vi "Configure Subnet Mask.vi"(0 "VISA resource name":refnum<visa-resource-name>, 5 "Subnet Mask (255.255.255.0)":string="255.255.255.0", 11 "error in (no error)":errorcluster) -> (4 "VISA resource name out":refnum<visa-resource-name>, 15 "error out":errorcluster)   [LabVIEW 2016, in "APT 300XAC Series.lvlib"]
doc: "Sets the Subnet Mask Of the APT 300xAC Series Power Source instrument"
uses:
  APT 300XAC Series.lvlib
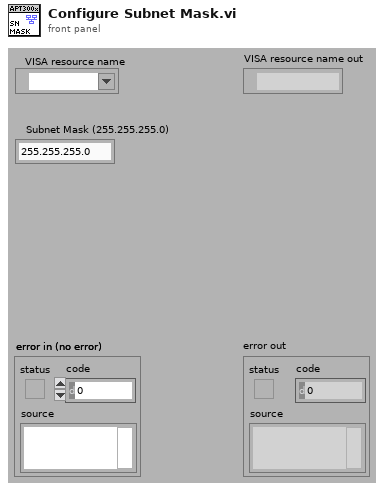
[diagram p1: front panel]
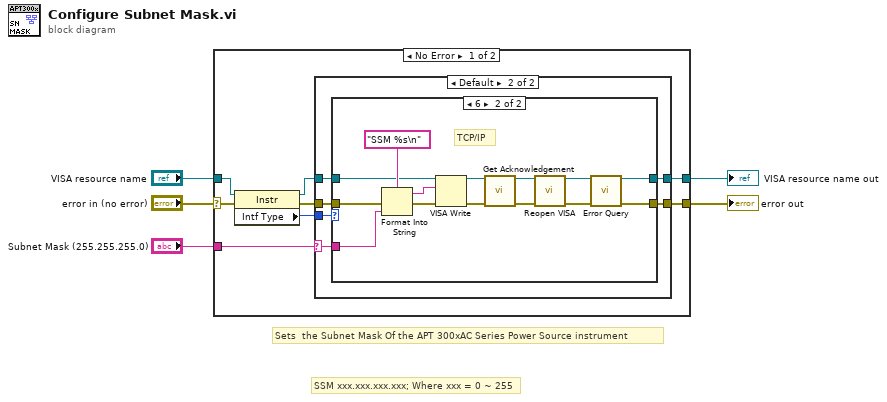
[diagram p0: block diagram]
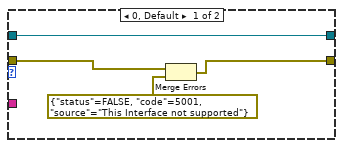
[diagram p3: hidden frame]
diagram:
  # "SSM xxx.xxx.xxx.xxx; Where xxx = 0 ~ 255"
  # "Sets  the Subnet Mask Of the APT 300xAC Series Power Source instrument"
  n1 = case shown="No Error" "error in (no error)" {
    selector: "error in (no error)" -> [w11 w41]
    tunnel: "VISA resource name" -> [w9 w40]
    tunnel: [w13 w40] -> w2
    tunnel: [w12 w41] -> w1
    tunnel: "Subnet Mask (255.255.255.0)" -> [w6 _]
    frame No Error {
      n2 = property class="Instr"(reference=w9, error in=w11) -> (reference out=w8:refnum<visa-resource-name>, error out=w10:errorcluster, "Intf Type"=w7:u16)
      n3 = case shown="Default" w6 {
        selector: w6 -> [_ w16]
        tunnel: [w15 w21] -> w13
        tunnel: [w14 w20] -> w12
        tunnel: w10 -> [w14 w19]
        tunnel: w8 -> [w15 w18]
        tunnel: w7 -> [_ w17]
        frame "" {
        }
        frame Default {
          n4 = case shown="6" w17 {
            tunnel: [w25 w39] -> w21
            tunnel: [w23 w37] -> w20
            tunnel: w16 -> [_ w33]
            tunnel: w19 -> [w22 w30]
            tunnel: w18 -> [w25 w29]
            frame 0, Default {
              n5 = Merge Errors(w22, errorcluster {"status"=FALSE, "code"=5001, "source"="This Interface not supported"} ("error in 2 (no error)")) -> (w23:errorcluster)
            }
            frame 6 {
              # "TCP/IP"
              n6 = Format Into String(format string="SSM %s\n" ("Command to Send"), error in=w30, w33) -> (resulting string=w36:string, error out=w35:errorcluster)  [unwired: 1 in]
              n7 = VISA Write(VISA resource name=w29, write buffer=w36, error in (no error)=w35) -> (VISA resource name out=w31:refnum<visa-resource-name>, error out=w38:errorcluster)  [unwired: 1 out]
              n8 = call "Get Acknowledgement.vi"("VISA resource name"=w31, "error in (no error)"=w38) -> ("VISA resource name out"=w27:refnum<visa-resource-name>, "error out"=w32:errorcluster)  [unwired: 12 in]
              n9 = call "Reopen VISA.vi"("VISA resource name"=w27, "error in (no error)"=w32) -> ("VISA resource name out"=w26:refnum<visa-resource-name>, "error out"=w28:errorcluster)  [unwired: 12 in]
              n10 = call "Error Query.vi"("VISA resource name"=w26, "error in (no error)"=w28) -> ("VISA resource name out"=w39:refnum<visa-resource-name>, "error out"=w37:errorcluster)  [unwired: 10 in, 2 out]
            }
          }
        }
      }
    }
    frame Error {
    }
  }
  "error out" <- w1
  "VISA resource name out" <- w2
